vi "Zusatzinformation test.vi"() -> ()   [LabVIEW 2010]
uses:
  <vilib>/regexp/Match Regular Expression.xnode
panel:
  out "Verknüpfter String":string
  in  "Numerisch 3":dbl
  in  "Numerisch 2":dbl
  in  "Numerisch":dbl
  out "Ausgabe-String":string
  in  "Regulärer Ausdruck":string
  in  "Stopp 2":bool
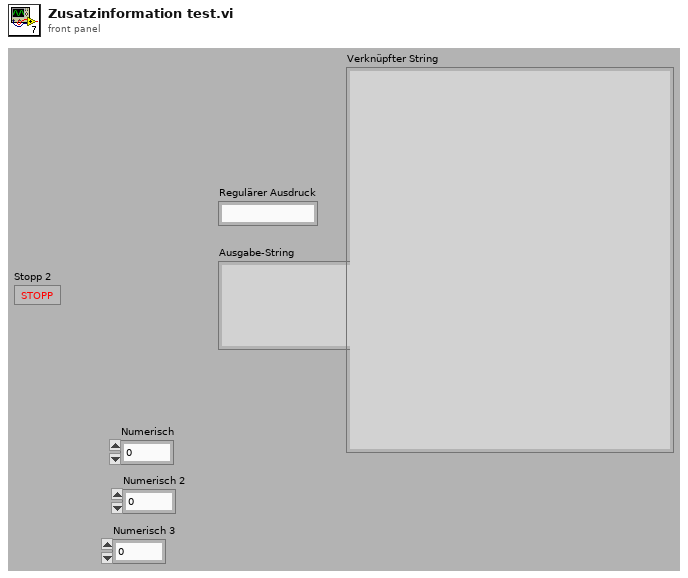
[diagram p1: front panel]
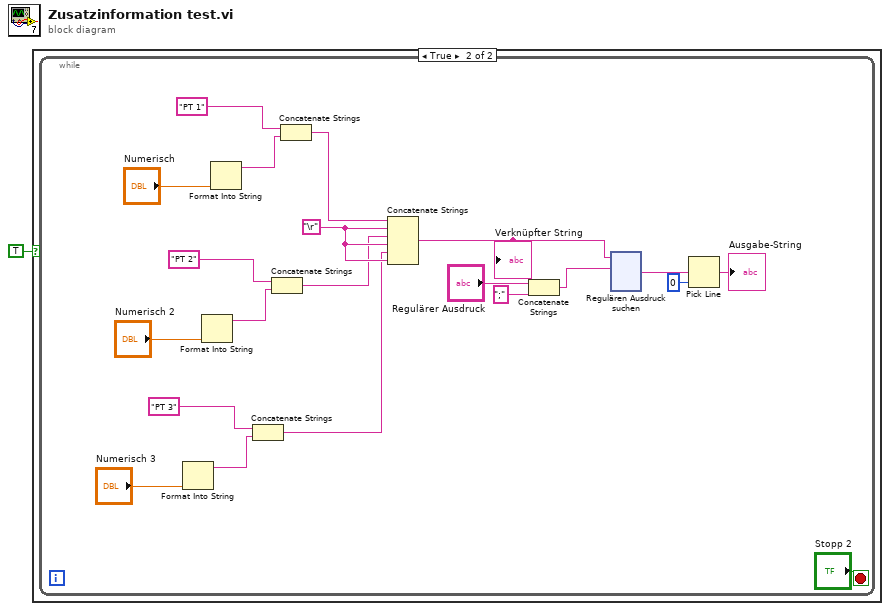
[diagram p0: block diagram]
diagram:
  n1 = case shown="True" TRUE {
    frame False {
    }
    frame True {
      n2 = while {
        stop <- "Stopp 2" stop-if-true
        w20 = "\r"
        n3 = Format Into String("Numerisch 3") -> (resulting string=w3:string)  [unwired: 3 in, 1 out]
        n4 = Format Into String("Numerisch 2") -> (resulting string=w2:string)  [unwired: 3 in, 1 out]
        n5 = Format Into String("Numerisch") -> (resulting string=w4:string)  [unwired: 3 in, 1 out]
        n6 = Concatenate Strings("PT 3" ("String"), w3) -> (w8:string)
        n7 = Concatenate Strings("PT 2" ("String"), w2) -> (w9:string)
        n8 = Concatenate Strings("PT 1" ("String"), w4) -> (w21:string)
        n9 = Concatenate Strings(w21, w20, w9, w20, w8, w20) -> (w19:string)
        "Verknüpfter String" <- w19
        n10 = Concatenate Strings("Regulärer Ausdruck", ";" ("String")) -> (w5:string)
        n11 = xnode "Regulären Ausdruck suchen"("Eingangs-String"=w19, "Regulärer Ausdruck"=w5) -> ("Nach Übereinstimmung"=w17:string)  [unwired: 4 in, 4 out]
        n12 = Pick Line(multi-line string=w17, line index=0 ("Zeilenindex")) -> (output string=→"Ausgabe-String":string)  [unwired: 1 in]
      }
    }
  }
